vi "Read Fixture ID.vi"(8 "error in (no error)":errorcluster, 11 "Fixture in":refnum<class "Fixture.lvclass">) -> (0 "error out":errorcluster, 2 "Fixture ID":i32, 3 "Fixture out":refnum<class "Fixture.lvclass">)   [LabVIEW 2019, in "Fixture.lvclass"]
uses:
  Fixture.lvclass
  Fixture.lvclass/Fixture.ctl
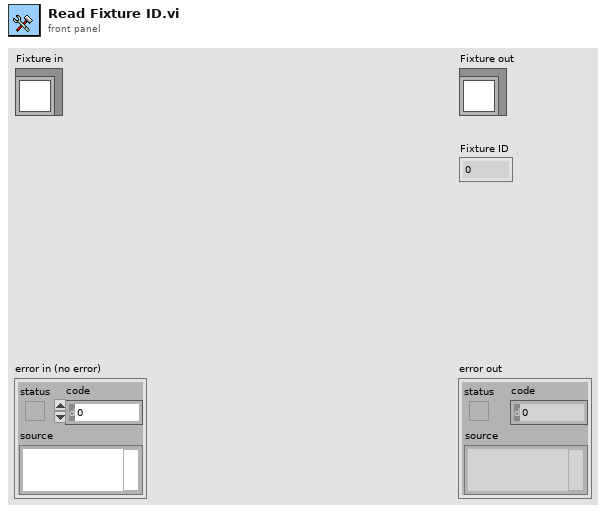
[diagram p1: front panel]
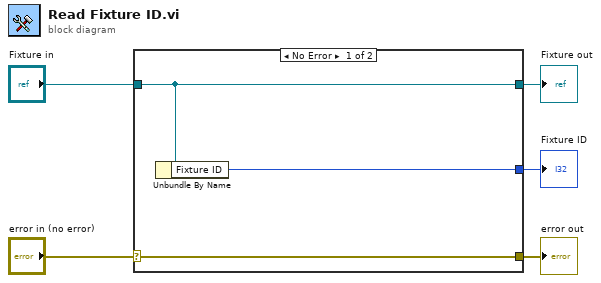
[diagram p0: block diagram]
diagram:
  n1 = case shown="No Error" "error in (no error)" {
    selector: "error in (no error)" -> [w8 w9]
    tunnel: [w8 w9] -> w4
    tunnel: [w7 w10] -> w2
    tunnel: "Fixture in" -> [w7 w10]
    tunnel: [w6 _] -> w1
    frame No Error {
      n2 = Unbundle By Name(w7) -> ("Fixture ID"=w6:i32)
    }
    frame Error {
    }
  }
  "error out" <- w4
  "Fixture out" <- w2
  "Fixture ID" <- w1
